vi "ReadTrackerResponse.vi"(8 "error in":errorcluster, 10 "timeout ms (1000)":i32, 11 "connection ID in":refnum<k5>) -> (0 "error out":errorcluster, 2 "Tracker Response":string, 3 "connection ID out":refnum<k5>)   [LabVIEW 2017]
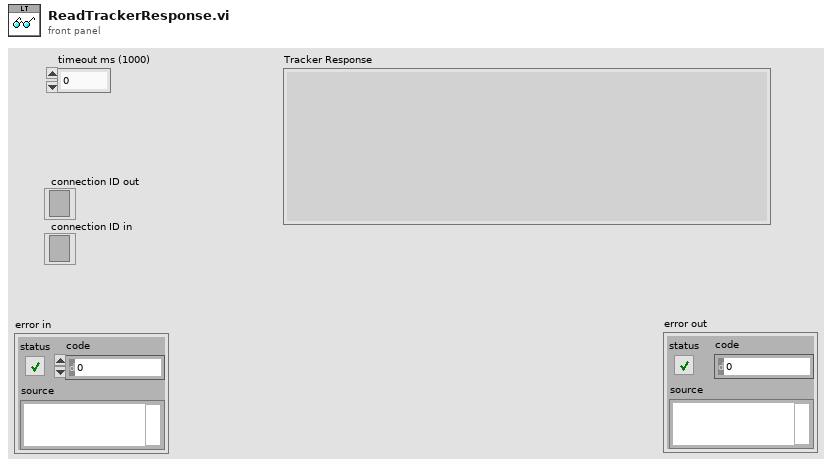
[diagram p1: front panel]
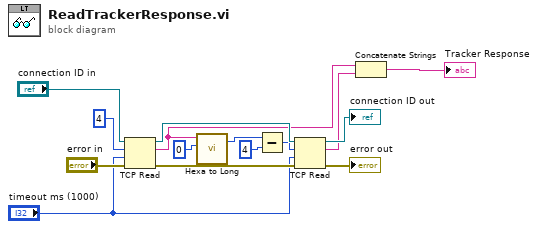
[diagram p0: block diagram]
diagram:
  n1 = TCP Read(connection ID="connection ID in", bytes to read=4, error in (no error)="error in", 9:"timeout ms (1000)") -> (connection ID out=w13:refnum<k5>, data out=w2:string, error out=w15:errorcluster)  [unwired: 1 in]
  n2 = call "Hexa to Long.vi"("Hexa"=w2, "Index"=0) -> ("Long"=w1:u32)  [unwired: 4 in]
  n3 = Subtract(x=w1, y=4 ("Index")) -> (x-y=w5:u32)
  n4 = TCP Read(connection ID=w13, bytes to read=w5, error in (no error)=w15, 9:"timeout ms (1000)") -> (connection ID out=→"connection ID out":refnum<k5>, data out=w4:string, error out=→"error out":errorcluster)  [unwired: 1 in]
  n5 = Concatenate Strings(w2, w4) -> (→"Tracker Response":string)
